vi "hidSPD Read Telemetry.vi"(8 "error in (no error)":errorcluster, 11 "spdDevSession in":T2 {"hidSPD.Sturtup Values"."HV_bias" format="%#_6p, V"; "hidSPD.Sturtup Values"."TSet" format="%#_6p, DegC"; "hidSPD.Controller"."HV_bias" format="%#_6p, V"; "hidSPD.Controller"."TSet" format="%#_6p, DegC"}) -> (0 "error out":errorcluster, 2 "telemetry":T1, 3 "spdDevSession out":T2 {"hidSPD.Sturtup Values"."HV_bias" format="%#_6p, V"; "hidSPD.Sturtup Values"."TSet" format="%#_6p, DegC"; "hidSPD.Controller"."HV_bias" format="%#_6p, V"; "hidSPD.Controller"."TSet" format="%#_6p, DegC"})   [LabVIEW 2018, in "hidSPDLibForLabView.lvlib"]
uses:
  hidSPDLibForLabView.lvlib
  hidSPD Controls/hidSPD Device Session.ctl
  hidSPD Controls/hidSPD Controller.ctl
  hidSPD Controls/hidSPD SPD Type.ctl
  hidSPD Controls/hidSPD Simple Report.ctl
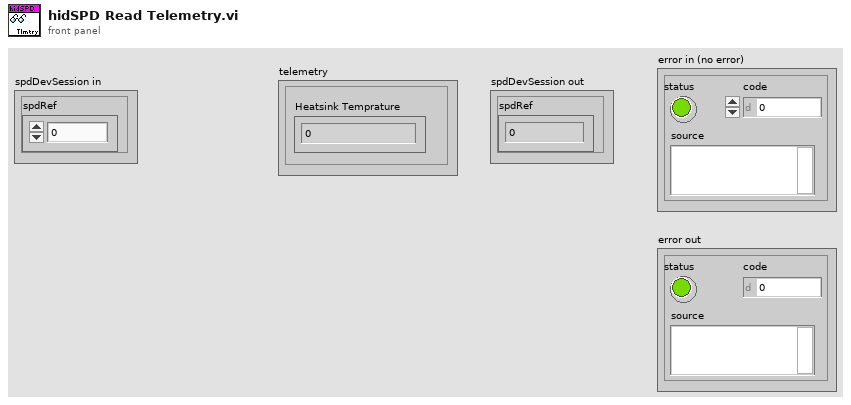
[diagram p1: front panel]
types:
  T1 = typedef "hidSPDLibForLabView.lvlib/hidSPD Simple Report.ctl" = cluster{"Heatsink Temprature":sgl, "Diod Temprature":sgl, "TEC-voltage":sgl, "Diod Bias":sgl, "RF Power":sgl, "Thrm_used":sgl, "hv_bias_used":sgl, "hv_code_used":u16, "stb_code_used":u16, "SPD number":u8, "SPD ready":u8, "status SPD":u32, "PLL_ErrorCount":u8, "Thrm_end":sgl, "stableI":sgl, "pid_error":sgl, "Bias_VD_Setpoint":sgl}
  T2 = typedef "hidSPDLibForLabView.lvlib/hidSPD Device Session.ctl" = cluster{"spdRef":u64, "connected":bool, "spdName":string, "hidSPD.Controller":T3, "hidSPD.Sturtup Values":T3, "SPD Type":T4}
  T3 = typedef "hidSPDLibForLabView.lvlib/hidSPD Controller.ctl" = cluster{"TSet":sgl, "HV_bias":sgl, "DDS_stb_code":u16}
  T4 = typedef "hidSPDLibForLabView.lvlib/hidSPD SPD Type.ctl" = enum16{"Free Run", "Strobe"}
  T5 = enum16{"big-endian, network order", "native, host order", "little-endian"}
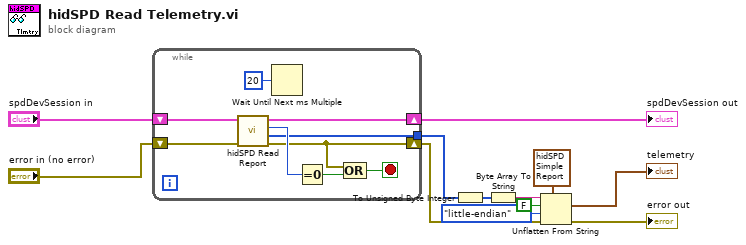
[diagram p0: block diagram]
diagram:
  n1 = while {
    shift-right: [w20] -> w11
    shift-left: "spdDevSession in" -> [w21]
    tunnel: [w16] -> w9
    shift-right: [w14] -> w4
    shift-left: "error in (no error)" -> [w19]
    stop <- w13 stop-if-true
    n2 = call "hidSPD Read Report.vi"("error in (no error)"=w19, "spdDevSession in"=w21) -> ("error out"=w14:errorcluster, "data"=w16:i32[], "cmd"=w17:i32, "spdDevSession out"=w20:T2)  [unwired: 6 in]
    n3 = Wait Until Next ms Multiple(millisecond multiple=u32 20) -> ()  [unwired: 1 out]
    n4 = Equal To 0?(x=w17) -> (x = 0?=w15:bool)
    n5 = Compound Arithmetic op=OR(w14, w15) -> (w13:bool)
  }
  "spdDevSession out" <- w11
  n6 = To Unsigned Byte Integer(number=w9) -> (unsigned 8bit integer=w8:u8[])
  n7 = Byte Array To String(unsigned byte array=w8) -> (string=w7:string)
  n8 = Unflatten From String(type=T1 {"Heatsink Temprature"=0.0, "Diod Temprature"=0.0, "TEC-voltage"=0.0, "Diod Bias"=0.0, "RF Power"=0.0, "Thrm_used"=0.0, "hv_bias_used"=0.0, "hv_code_used"=0, "stb_code_used"=0, "SPD number"=0, "SPD ready"=0, "status SPD"=0, "PLL_ErrorCount"=0, "Thrm_end"=0.0, "stableI"=0.0, "pid_error"=0.0, "Bias_VD_Setpoint"=0.0} ("hidSPD Simple Report"), binary string=w7, data includes array or string size? (T)=FALSE, byte order (0:big-endian, network order)=T5."little-endian", error in (no error)=w4) -> (value=→"telemetry":T1, error out=→"error out":errorcluster)  [unwired: 1 out]
